vi "Swerve Math.vi"(0 "Gyro":dbl, 1 "FWD":dbl(slide) scale=-1.0..1.0, 2 "STR":dbl(slide) scale=-1.0..1.0, 3 "RCW":dbl(slide) scale=-1.0..1.0) -> (7 "Wheel Speeds":dbl[](array[numeric]), 9 "Wheel Angles":dbl[](array[numeric]))   [LabVIEW 2020]
panel:
  in  "Gyro Working":bool=TRUE
  out "STR(Field)":dbl
  out "FWD(Field)":dbl
  out "MAX(before normalized)":dbl
  out "WA 4":dbl
  out "WA 3":dbl
  out "WA 2":dbl
  out "WA 1":dbl
  out "WS 4":dbl
  out "WS 3":dbl
  out "WS 2":dbl
  out "WS 1":dbl
  out "D":dbl
  out "C":dbl
  out "B":dbl
  out "A":dbl
  in  "Width(Left to Right)":dbl=30.0
  in  "Length(Front to Back)":dbl=24.0
  # "From the Center of the Wheels"
  # "Forward/Back"
  # "Left/Right"
  # "Rotation(Clockwise)"
  # "Units are irrelevant"
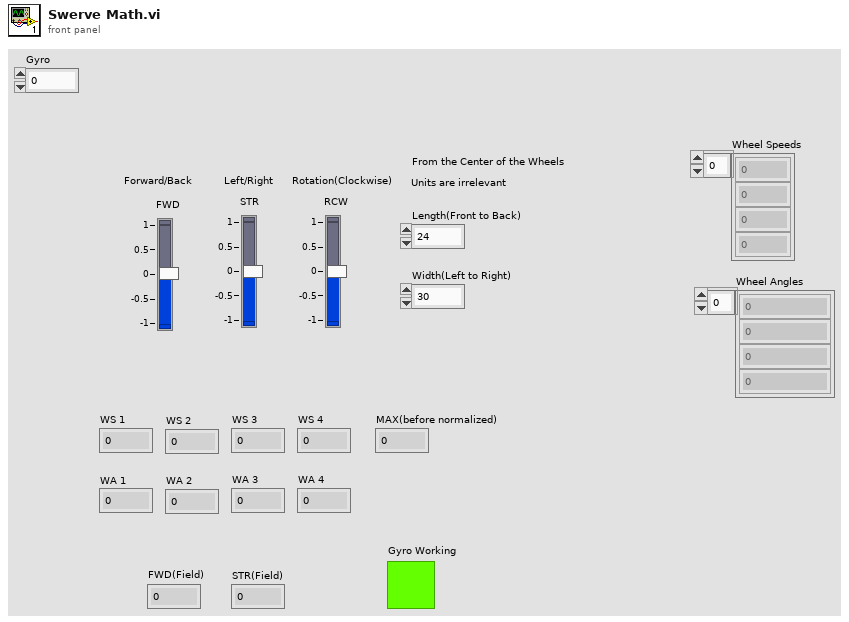
[diagram p1: front panel]
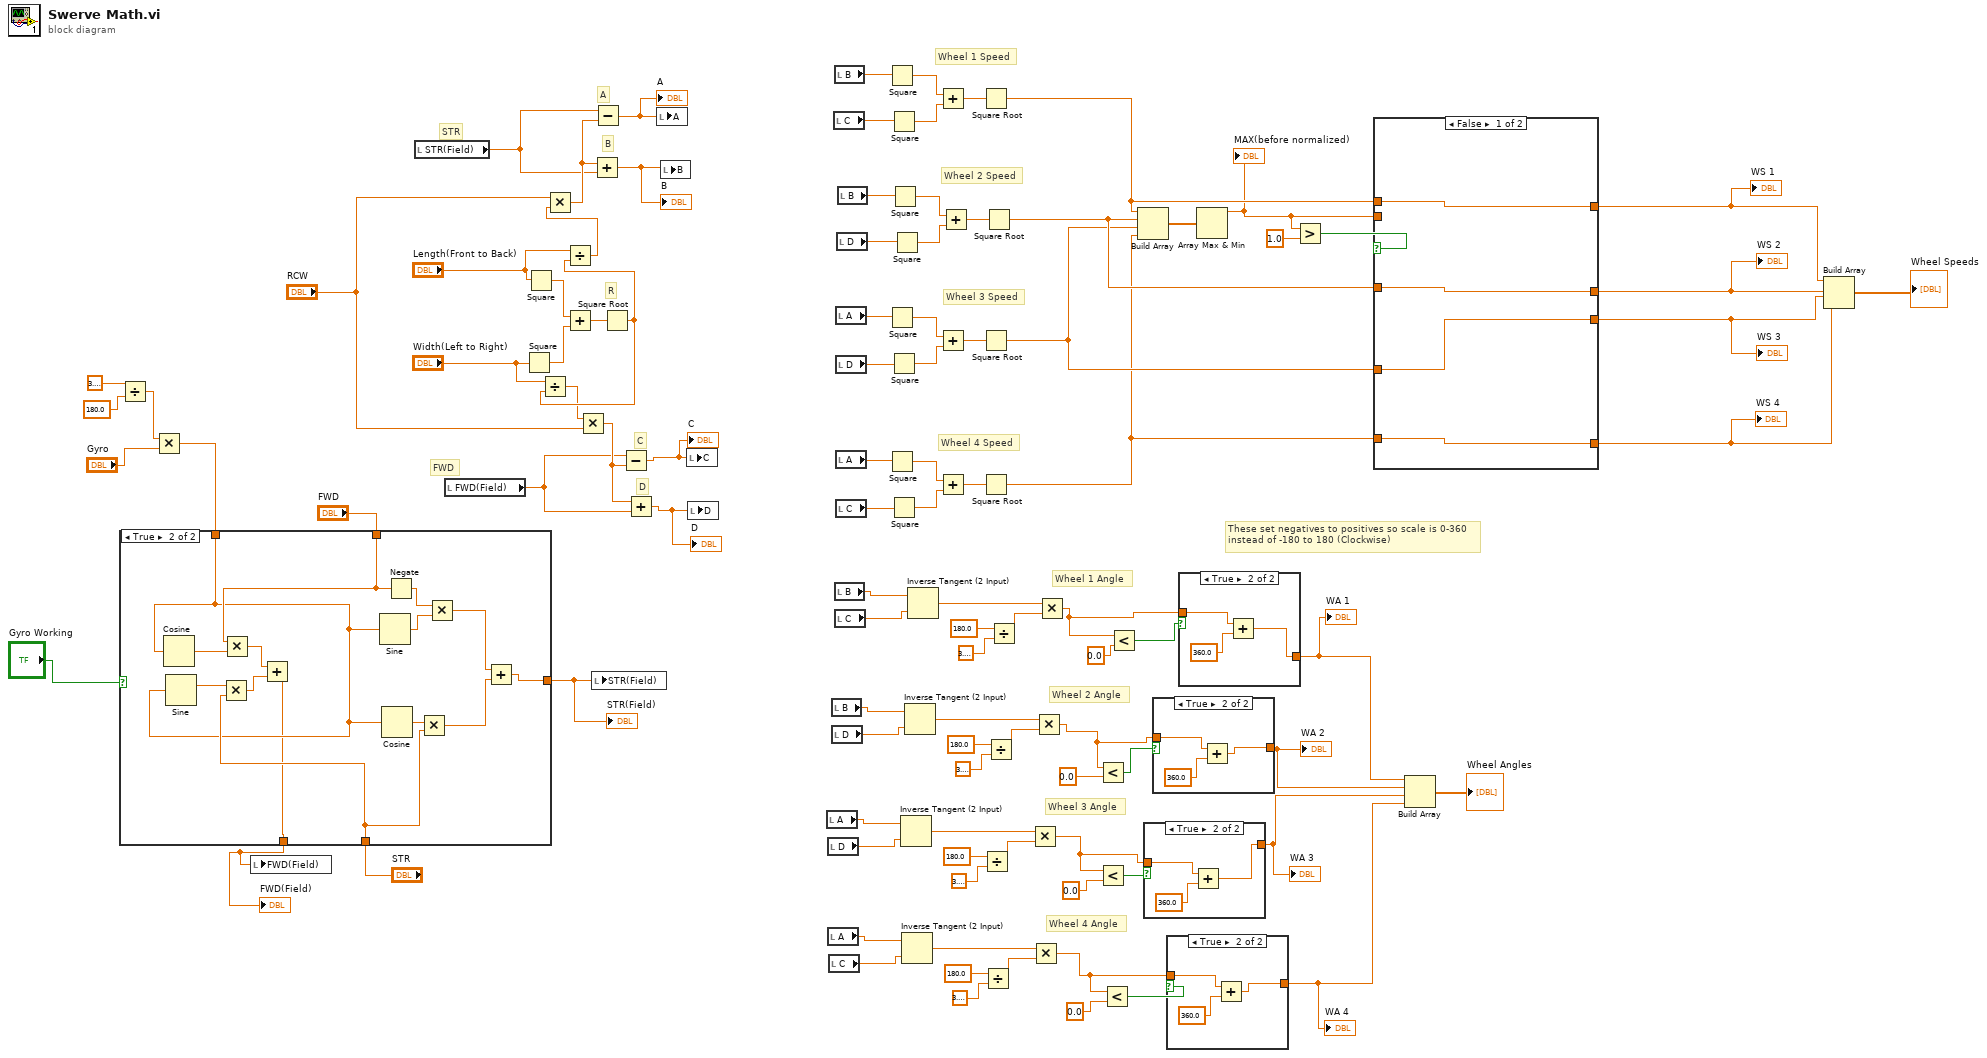
[diagram p0: block diagram]
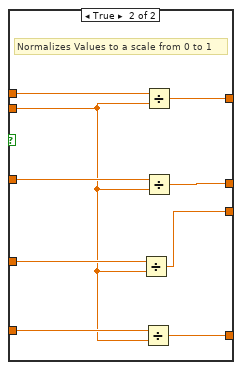
[diagram p2: hidden frame]
diagram:
  # "These set negatives to positives so scale is 0-360\ninstead of -180 to 180 (Clockwise)"
  # "FWD"
  # "STR"
  # "Wheel 4 Angle"
  # "Wheel 3 Angle"
  # "Wheel 2 Angle"
  # "Wheel 1 Angle"
  # "Wheel 4 Speed"
  # "Wheel 3 Speed"
  # "Wheel 2 Speed"
  # "Wheel 1 Speed"
  # "D"
  # "C"
  # "B"
  # "A"
  # "R"
  n1 = Divide(x=3.141592653589793, y=180.0 ("x")) -> (x/y=w26:dbl)
  n2 = Multiply(x=w26, y="Gyro") -> (x*y=w25:dbl)
  n3 = case shown="True" "Gyro Working" {
    tunnel: "STR" -> [w103 w108]
    tunnel: "FWD" -> [w102 w107]
    tunnel: [w103 w106] -> w34
    tunnel: w25 -> [_ w105]
    tunnel: [w102 w104] -> w33
    frame False {
    }
    frame True {
      n4 = Cosine(x=w105) -> (cos(x)=w109:dbl)
      n5 = Sine(x=w105) -> (sin(x)=w110:dbl)
      n6 = Multiply(x=w110, y=w108) -> (x*y=w111:dbl)
      n7 = Multiply(x=w107, y=w109) -> (x*y=w112:dbl)
      n8 = Add(x=w112, y=w111) -> (x+y=w104:dbl)
      n9 = Sine(x=w105) -> (sin(x)=w117:dbl)
      n10 = Cosine(x=w105) -> (cos(x)=w116:dbl)
      n11 = Negate(x=w107) -> (-x=w115:dbl)
      n12 = Multiply(x=w116, y=w108) -> (x*y=w114:dbl)
      n13 = Multiply(x=w115, y=w117) -> (x*y=w113:dbl)
      n14 = Add(x=w113, y=w114) -> (x+y=w106:dbl)
    }
  }
  "STR(Field)" <- w34
  "FWD(Field)" <- w33
  n15 = local write "FWD(Field)"(w33) -> ()
  n16 = local read "STR(Field)"() -> (w31:dbl)
  n17 = local read "FWD(Field)"() -> (w32:dbl)
  n18 = Square(x="Width(Left to Right)") -> (x^2=w99:dbl)
  n19 = Square(x="Length(Front to Back)") -> (x^2=w100:dbl)
  n20 = Add(x=w100, y=w99) -> (x+y=w101:dbl)
  n21 = local write "STR(Field)"(w34) -> ()
  n22 = Square Root(x=w101) -> (sqrt(x)=w97:dbl)
  n23 = Divide(x="Width(Left to Right)", y=w97) -> (x/y=w93:dbl)
  n24 = Divide(x="Length(Front to Back)", y=w97) -> (x/y=w95:dbl)
  n25 = Multiply(x="RCW", y=w95) -> (x*y=w92:dbl)
  n26 = Multiply(x=w93, y="RCW") -> (x*y=w91:dbl)
  n27 = Add(x=w92, y=w31) -> (x+y=w90:dbl)
  "B" <- w90
  n28 = Subtract(x=w31, y=w92) -> (x-y=w89:dbl)
  "A" <- w89
  n29 = Subtract(x=w32, y=w91) -> (x-y=w87:dbl)
  "C" <- w87
  n30 = Add(x=w91, y=w32) -> (x+y=w88:dbl)
  "D" <- w88
  n31 = local write "A"(w89) -> ()
  n32 = local write "B"(w90) -> ()
  n33 = local write "C"(w87) -> ()
  n34 = local write "D"(w88) -> ()
  n35 = local read "A"() -> (w45:dbl)
  n36 = local read "D"() -> (w44:dbl)
  n37 = local read "A"() -> (w39:dbl)
  n38 = local read "C"() -> (w38:dbl)
  n39 = local read "B"() -> (w51:dbl)
  n40 = local read "D"() -> (w50:dbl)
  n41 = local read "C"() -> (w83:dbl)
  n42 = local read "B"() -> (w82:dbl)
  n43 = local read "B"() -> (w57:dbl)
  n44 = local read "C"() -> (w56:dbl)
  n45 = local read "A"() -> (w73:dbl)
  n46 = local read "D"() -> (w72:dbl)
  n47 = local read "A"() -> (w68:dbl)
  n48 = local read "C"() -> (w67:dbl)
  n49 = local read "D"() -> (w78:dbl)
  n50 = local read "B"() -> (w77:dbl)
  n51 = Square(x=w82) -> (x^2=w84:dbl)
  n52 = Square(x=w73) -> (x^2=w74:dbl)
  n53 = Square(x=w68) -> (x^2=w69:dbl)
  n54 = Square(x=w83) -> (x^2=w85:dbl)
  n55 = Square(x=w72) -> (x^2=w75:dbl)
  n56 = Square(x=w67) -> (x^2=w70:dbl)
  n57 = Square(x=w77) -> (x^2=w79:dbl)
  n58 = Square(x=w78) -> (x^2=w80:dbl)
  n59 = Inverse Tangent (2 Input)(1:w44, 2:w45) -> (0:w49:dbl)
  n60 = Inverse Tangent (2 Input)(1:w38, 2:w39) -> (0:w43:dbl)
  n61 = Inverse Tangent (2 Input)(1:w50, 2:w51) -> (0:w55:dbl)
  n62 = Inverse Tangent (2 Input)(1:w56, 2:w57) -> (0:w61:dbl)
  n63 = Add(x=w84, y=w85) -> (x+y=w86:dbl)
  n64 = Add(x=w74, y=w75) -> (x+y=w76:dbl)
  n65 = Add(x=w69, y=w70) -> (x+y=w71:dbl)
  n66 = Add(x=w79, y=w80) -> (x+y=w81:dbl)
  n67 = Square Root(x=w86) -> (sqrt(x)=w64:dbl)
  n68 = Square Root(x=w76) -> (sqrt(x)=w63:dbl)
  n69 = Square Root(x=w71) -> (sqrt(x)=w62:dbl)
  n70 = Divide(x=180.0, y=3.141592653589793) -> (x/y=w48:dbl)
  n71 = Divide(x=180.0, y=3.141592653589793) -> (x/y=w42:dbl)
  n72 = Square Root(x=w81) -> (sqrt(x)=w65:dbl)
  n73 = Divide(x=180.0, y=3.141592653589793) -> (x/y=w54:dbl)
  n74 = Divide(x=180.0, y=3.141592653589793) -> (x/y=w60:dbl)
  n75 = Multiply(x=w49, y=w48) -> (x*y=w12:dbl)
  n76 = Multiply(x=w43, y=w42) -> (x*y=w14:dbl)
  n77 = Multiply(x=w55, y=w54) -> (x*y=w15:dbl)
  n78 = Multiply(x=w61, y=w60) -> (x*y=w16:dbl)
  n79 = Less?(x=w15, y=0.0) -> (x < y?=w17:bool)
  n80 = Less?(x=w12, y=0.0) -> (x < y?=w19:bool)
  n81 = Less?(x=w14, y=0.0) -> (x < y?=w22:bool)
  n82 = Less?(x=w16, y=0.0) -> (x < y?=w23:bool)
  n83 = Build Array(w64, w65, w63, w62) -> (w66:dbl[])
  n84 = case shown="True" w19 {
    tunnel: w12 -> [w118 w120]
    tunnel: [w118 w119] -> w11
    frame False {
    }
    frame True {
      n85 = Add(x=w120, y=360.0) -> (x+y=w119:dbl)
    }
  }
  "WA 3" <- w11
  n86 = case shown="True" w17 {
    tunnel: w15 -> [w122 w124]
    tunnel: [w122 w123] -> w13
    frame False {
    }
    frame True {
      n87 = Add(x=w124, y=360.0) -> (x+y=w123:dbl)
    }
  }
  "WA 2" <- w13
  n88 = case shown="True" w22 {
    tunnel: w14 -> [w126 w128]
    tunnel: [w126 w127] -> w9
    frame False {
    }
    frame True {
      n89 = Add(x=w128, y=360.0) -> (x+y=w127:dbl)
    }
  }
  "WA 4" <- w9
  n90 = case shown="True" w23 {
    tunnel: w16 -> [w130 w132]
    tunnel: [w130 w131] -> w10
    frame False {
    }
    frame True {
      n91 = Add(x=w132, y=360.0) -> (x+y=w131:dbl)
    }
  }
  "WA 1" <- w10
  n92 = Array Max & Min(array=w66) -> (max value=w7:dbl)  [unwired: 3 out]
  "MAX(before normalized)" <- w7
  n93 = Greater?(x=w7, y=1.0) -> (0:w6:bool)
  n94 = case shown="False" w6 {
    tunnel: w65 -> [w136 w146]
    tunnel: w64 -> [w137 w145]
    tunnel: w63 -> [w135 w144]
    tunnel: w62 -> [w134 w143]
    tunnel: w7 -> [_ w142]
    tunnel: [w137 w141] -> w4
    tunnel: [w136 w140] -> w3
    tunnel: [w135 w139] -> w2
    tunnel: [w134 w138] -> w1
    frame False {
    }
    frame True {
      # "Normalizes Values to a scale from 0 to 1"
      n95 = Divide(x=w144, y=w142) -> (x/y=w139:dbl)
      n96 = Divide(x=w143, y=w142) -> (x/y=w138:dbl)
      n97 = Divide(x=w145, y=w142) -> (x/y=w141:dbl)
      n98 = Divide(x=w146, y=w142) -> (x/y=w140:dbl)
    }
  }
  "WS 1" <- w4
  "WS 2" <- w3
  "WS 3" <- w2
  "WS 4" <- w1
  n99 = Build Array(w10, w13, w11, w9) -> (→"Wheel Angles":dbl[])
  n100 = Build Array(w4, w3, w2, w1) -> (→"Wheel Speeds":dbl[])
